vi "ErrorDrawerConfig.vi"(8 "Error In":errorcluster) -> (0 "Error Out":errorcluster)   [LabVIEW 2017, in "ErrorStructureDrawer.lvlib"]
doc: "Hardcoded config settings are stored here. The developer using the error structure drawer tool may edit these settings if desired.\n\nE.g. the developer may change spacings between various elements, error cluster style, or alignment of items."
uses:
  ErrorStructureDrawer.lvlib
  Controls/CaseStructureOuterWhitespace.ctl
  Controls/CaseStructureInnerWhitespace.ctl
  Controls/CaseStructureConstants.ctl
  Controls/ErrorControlConfig.ctl
  Controls/ErrorControlType.ctl
  Controls/BD_AlignmentSettings.ctl
  Controls/ErrorStructureDrawerSettings.ctl
  Controls/CaseStructureSizeIfBD_Empty.ctl
  Controls/ControlConstants.ctl
  Controls/GetSetCommand.ctl
  Controls/ControlIndicatorAlignment.ctl
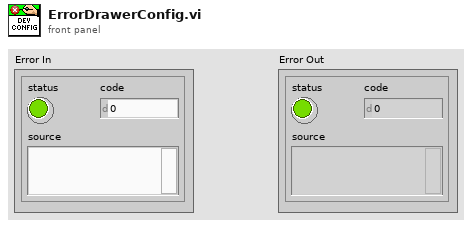
[diagram p1: front panel]
types:
  T1 = typedef "ErrorStructureDrawer.lvlib/ControlIndicatorAlignment.ctl" = enum32{"Top Edges", "Vertical Centers", "Bottom Edges", "Left Edges", "Horizontal Centers", "Right Edges", "Auto"}
  T2 = typedef "ErrorStructureDrawer.lvlib/ControlConstants.ctl" = cluster{"Half-height of terminal":i32}
  T3 = typedef "ErrorStructureDrawer.lvlib/ErrorControlType.ctl" = enum16{"Silver", "Modern", "Classic", "LabVIEW default"}
  T4 = typedef "ErrorStructureDrawer.lvlib/CaseStructureSizeIfBD_Empty.ctl" = cluster{"Width (%)":dbl, "Height (%)":dbl}
  T5 = typedef "ErrorStructureDrawer.lvlib/GetSetCommand.ctl" = enum16{"Get", "Set"}
  T6 = typedef "ErrorStructureDrawer.lvlib/ErrorStructureDrawerSettings.ctl" = cluster{"Error control config":T7, "BD alignment settings":T8, "Case structure outer whitespace (px)":T9, "Case structure inner whitespace (px)":T10, "Case structure constants":T11, "CS size if BD is empty":T4, "Control constants":T2}
  T7 = typedef "ErrorStructureDrawer.lvlib/ErrorControlConfig.ctl" = cluster{"Error control path":path, "Error indicator path":path, "Error control vertical spacing from existing FP items":i16, "Error-control to error-indicator horizontal spacing on FP":i16, "Error control vertical spacing from existing BD items":i32, "Error indicator vertical spacing from existing BD items":i32}
  T8 = typedef "ErrorStructureDrawer.lvlib/BD_AlignmentSettings.ctl" = cluster{"Controls":enum32{"Top Edges", "Vertical Centers", "Bottom Edges", "Left Edges", "Horizontal Centers", "Right Edges"}, "Indicators":enum32{"Top Edges", "Vertical Centers", "Bottom Edges", "Left Edges", "Horizontal Centers", "Right Edges"}}
  T9 = typedef "ErrorStructureDrawer.lvlib/CaseStructureOuterWhitespace.ctl" = cluster{"Control terminals right-side":i32, "Indicator terminals left-side":i32}
  T10 = typedef "ErrorStructureDrawer.lvlib/CaseStructureInnerWhitespace.ctl" = cluster{"Left":u32, "Right":u32, "Top":u32, "Bottom":u32}
  T11 = typedef "ErrorStructureDrawer.lvlib/CaseStructureConstants.ctl" = cluster{"Border thickness":u32, "Case-menu height":u32, "Half height/width of a tunnel":i32}
  T12 = enum32{"Top Edges", "Vertical Centers", "Bottom Edges", "Left Edges", "Horizontal Centers", "Right Edges"}
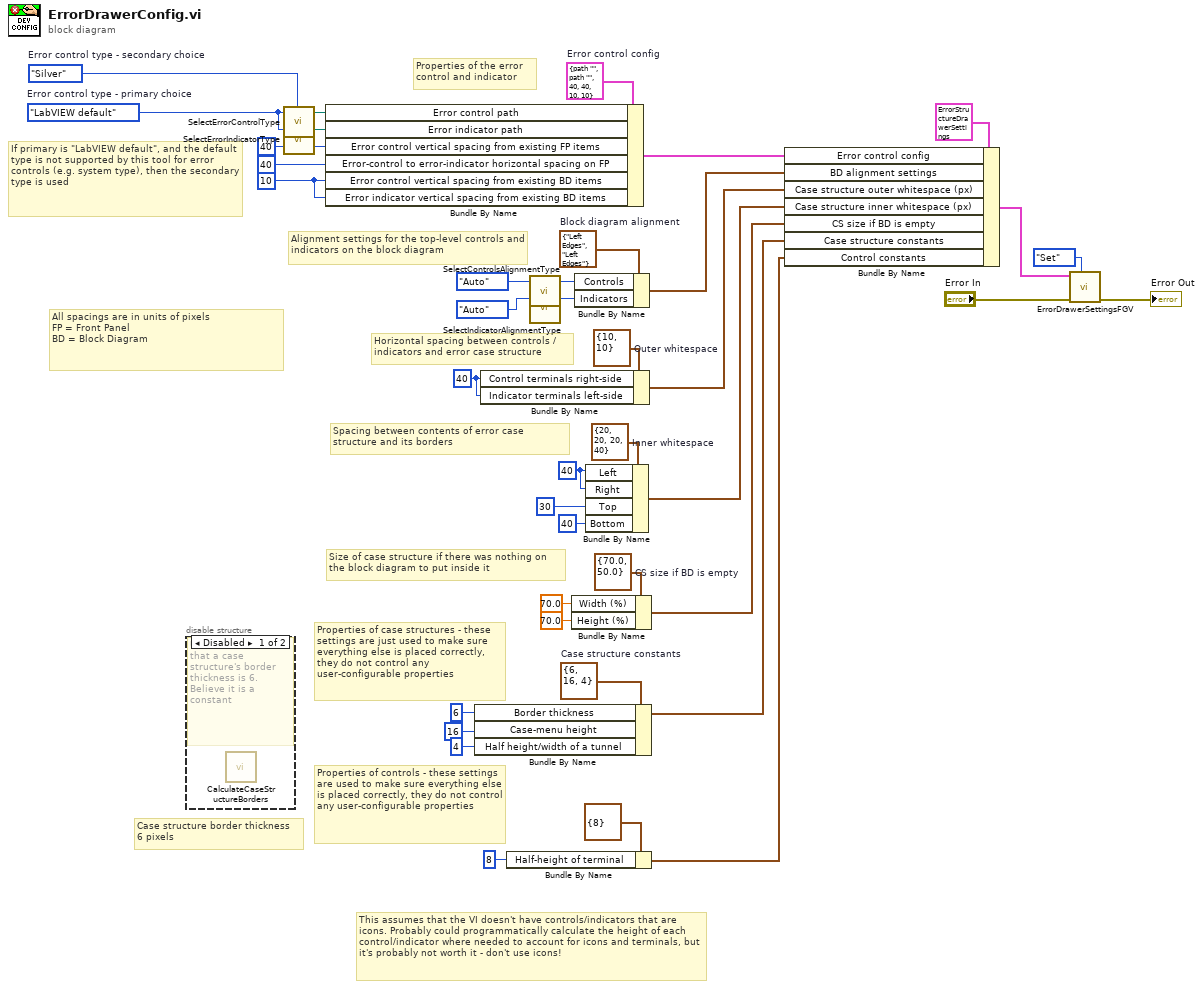
[diagram p0: block diagram]
diagram:
  w10 = ErrorControlType."Silver"  # Error control type - secondary choice
  w14 = T4 {"Width (%)"=70.0, "Height (%)"=50.0}  # CS size if BD is empty
  w28 = T8 {"Controls"=enum."Left Edges", "Indicators"=enum."Left Edges"}  # Block diagram alignment
  w18 = 10 ("Error control vertical spacing from existing BD controls")
  w29 = ErrorControlType."LabVIEW default"  # Error control type - primary choice
  w34 = T7 {"Error control path"=path "", "Error indicator path"=path "", "Error control vertical spacing from existing FP items"=40, "Error-control to error-indicator horizontal spacing on FP"=40, "Error control vertical spacing from existing BD items"=10, "Error indicator vertical spacing from existing BD items"=10}  # Error control config
  w17 = 40 ("Control terminals right-side")
  w16 = u32 40 ("Left")
  w39 = T11 {"Border thickness"=6, "Case-menu height"=16, "Half height/width of a tunnel"=4}  # Case structure constants
  w40 = T10 {"Left"=20, "Right"=20, "Top"=20, "Bottom"=40}  # Inner whitespace
  w38 = T9 {"Control terminals right-side"=10, "Indicator terminals left-side"=10}  # Outer whitespace
  # "This assumes that the VI doesn't have controls/indicators that are icons. Probably could programmatically calculate the height of each control/indicator where needed to account for icons and terminals, but it's probably not worth it - don't use icons!"
  # "Properties of controls - these settings are used to make sure everything else is placed correctly, they do not control any user-configurable properties"
  # "If primary is \"LabVIEW default\", and the default type is not supported by this tool for error controls (e.g. system type), then the secondary type is used"
  # "Size of case structure if there was nothing on the block diagram to put inside it"
  # "All spacings are in units of pixels\nFP = Front Panel\nBD = Block Diagram"
  # "Alignment settings for the top-level controls and indicators on the block diagram"
  # "Properties of the error control and indicator"
  # "Properties of case structures - these settings are just used to make sure everything else is placed correctly, they do not control any user-configurable properties"
  # "Spacing between contents of error case structure and its borders"
  # "Horizontal spacing between controls / indicators and error case structure"
  # "Case structure border thickness\n6 pixels"
  n1 = disable-structure shown="Disabled" {
    frame Disabled {
      # "Used this to find that a case structure's border thickness is 6. Believe it is a constant"
      n2 = call "CalculateCaseStructureBorders.vi"() -> ()  [unwired: 11 in, 1 out]
    }
    frame Enabled {
    }
  }
  n3 = call "SelectErrorControlType.vi"("Error control type (primary)"=w29, "Error control type (secondary)"=w10) -> ("Error control path"=w31:path)  [unwired: 25 in]
  n4 = call "SelectErrorIndicatorType.vi"("Error indicator type (primary)"=w29, "Error indicator type (secondary)"=w10) -> ("Error indicator path"=w30:path)  [unwired: 25 in]
  n5 = Bundle By Name(cluster=w34, "Error control path"=w31, "Error indicator path"=w30, "Error control vertical spacing from existing FP items"=i16 40 ("Error control vertical spacing from existing items"), "Error-control to error-indicator horizontal spacing on FP"=i16 40 ("Error-control to error-indicator horizontal spacing"), "Error control vertical spacing from existing BD items"=w18, "Error indicator vertical spacing from existing BD items"=w18) -> (w27:T7)
  n6 = Bundle By Name(cluster=w39, "Border thickness"=u32 6, "Case-menu height"=u32 16, "Half height/width of a tunnel"=4 ("Half height/width of a case structure tunnel")) -> (w15:T11)
  n7 = Bundle By Name(cluster=w38, "Control terminals right-side"=w17, "Indicator terminals left-side"=w17) -> (w25:T9)
  n8 = Bundle By Name(cluster=T2 {"Half-height of terminal"=8} ("Control constants"), "Half-height of terminal"=8 ("Half height of a control terminal")) -> (w5:T2)
  n9 = call "SelectControlsAlignmentType.vi"("Controls alignment type"=ControlIndicatorAlignment."Auto") -> ("Controls alignment type"=w4:T12)  [unwired: 26 in]
  n10 = call "SelectIndicatorAlignmentType.vi"("Indicators alignment type"=ControlIndicatorAlignment."Auto" ("Controls alignment type")) -> ("Indicators alignment type"=w3:T12)  [unwired: 26 in]
  n11 = Bundle By Name(cluster=w14, "Width (%)"=70.0, "Height (%)"=70.0) -> (w13:T4)
  n12 = Bundle By Name(cluster=w28, "Controls"=w4, "Indicators"=w3) -> (w26:T8)
  n13 = Bundle By Name(cluster=w40, "Left"=w16, "Right"=w16, "Top"=u32 30, "Bottom"=u32 40) -> (w24:T10)
  n14 = Bundle By Name(cluster=T6 {"Error control config"={"Error control path"=path "", "Error indicator path"=path "", "Error control vertical spacing from existing FP items"=40, "Error-control to error-indicator horizontal spacing on FP"=40, "Error control vertical spacing from existing BD items"=10, "Error indicator vertical spacing from existing BD items"=10}, "BD alignment settings"={"Controls"=enum."Left Edges", "Indicators"=enum."Left Edges"}, "Case structure outer whitespace (px)"={"Control terminals right-side"=10, "Indicator terminals left-side"=10}, "Case structure inner whitespace (px)"={"Left"=20, "Right"=20, "Top"=20, "Bottom"=40}, "Case structure constants"={"Border thickness"=6, "Case-menu height"=16, "Half height/width of a tunnel"=4}, "CS size if BD is empty"={"Width (%)"=70.0, "Height (%)"=50.0}, "Control constants"={"Half-height of terminal"=8}} ("Error structure drawer settings"), "Error control config"=w27, "BD alignment settings"=w26, "Case structure outer whitespace (px)"=w25, "Case structure inner whitespace (px)"=w24, "CS size if BD is empty"=w13, "Case structure constants"=w15, "Control constants"=w5) -> (w22:T6)
  n15 = call "ErrorDrawerSettingsFGV.vi"("Get or Set (Get)"=GetSetCommand."Set", "Error In"="Error In", "Error structure drawer settings"=w22) -> ("Error Out"=→"Error Out":errorcluster)  [unwired: 7 in, 1 out]
